vi "Get Image SGL Array.vi"(8 "error in (no error)":errorcluster, 11 "Refnum in":T1) -> (0 "error out":errorcluster, 3 "Pixel Array":sgl[][](array[numeric]))   [LabVIEW 2021, in "Image.lvlib"]
uses:
  <vilib>/vision/Image Controls.llb/IMAQ Image.ctl
  <vilib>/Utility/error.llb/Error Cluster From Error Code.vi
  <vilib>/ErrorRing/Error Ring.xnode
  Image.lvlib
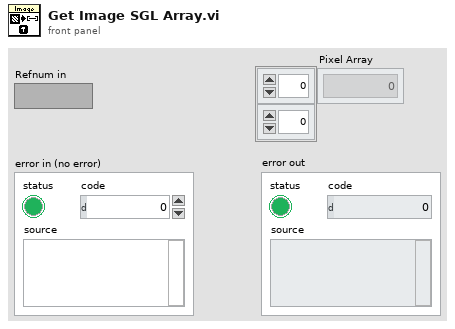
[diagram p1: front panel]
types:
  T1 = typedef "IMAQ Image.ctl" = refnum<image>
  T2 = typedef "Image Type" = u32
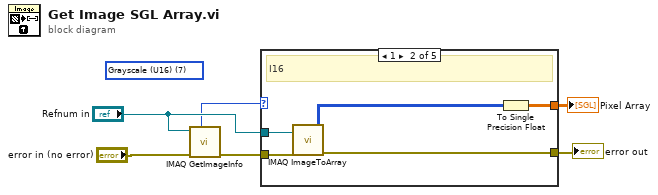
[diagram p0: block diagram]
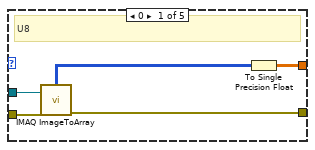
[diagram p2: hidden frame]
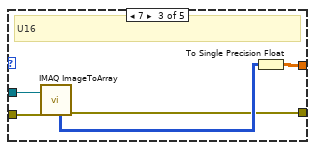
[diagram p3: hidden frame]
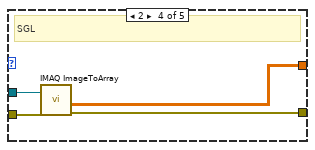
[diagram p4: hidden frame]
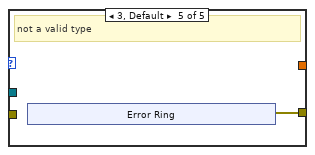
[diagram p5: hidden frame]
diagram:
  (unwired) T2 7 items=["Grayscale (U8)", "Grayscale (I16)", "Grayscale (SGL)", "Complex (CSG)", "RGB (U32)", "HSL (U32)", "RGB (U64)", "Grayscale (U16)"] ("Image Type")
  n1 = call "IMAQ GetImageInfo"("error in (no error)"="error in (no error)", "Image"="Refnum in") -> ("error out"=w4:errorcluster, "Image Type"=w3:T2)  [unwired: 2 in, 6 out]
  n2 = case shown="1" w3 {
    tunnel: "Refnum in" -> [w11 w16 w21 w25 _]
    tunnel: w4 -> [w10 w15 w20 w24 _]
    tunnel: [w8 w14 w19 w23 _] -> w2
    tunnel: [w7 w12 w17 w22 w26] -> w1
    frame 0 {
      # "U8"
      n3 = call "IMAQ ImageToArray"("error in (no error)"=w10, "Image"=w11) -> ("error out"=w7:errorcluster, "Image Pixels (U8)"=w9:u8[][])  [unwired: 2 in, 3 out]
      n4 = To Single Precision Float(number=w9) -> (single precision float=w8:sgl[][])
    }
    frame 1 {
      # "I16"
      n5 = call "IMAQ ImageToArray"("error in (no error)"=w15, "Image"=w16) -> ("error out"=w12:errorcluster, "Image Pixels (I16)"=w13:i16[][])  [unwired: 2 in, 3 out]
      n6 = To Single Precision Float(number=w13) -> (single precision float=w14:sgl[][])
    }
    frame 7 {
      # "U16"
      n7 = call "IMAQ ImageToArray"("error in (no error)"=w20, "Image"=w21) -> ("Image Pixels (U16)"=w18:u16[][], "error out"=w17:errorcluster)  [unwired: 2 in, 3 out]
      n8 = To Single Precision Float(number=w18) -> (single precision float=w19:sgl[][])
    }
    frame 2 {
      # "SGL"
      n9 = call "IMAQ ImageToArray"("error in (no error)"=w24, "Image"=w25) -> ("Image Pixels (Float)"=w23:sgl[][], "error out"=w22:errorcluster)  [unwired: 2 in, 3 out]
    }
    frame 3, Default {
      # "not a valid type"
      n10 = xnode "Error Ring"() -> ("error out"=w26:errorcluster)
    }
  }
  "Pixel Array" <- w2
  "error out" <- w1
